vi "ConvertStringToArmSource.vi"(11 "Arm Source String":string) -> (3 "Arm Source":T1)   [LabVIEW 2012, in "Keithley-7001.lvlib"]
uses:
  Keithley-7001.lvlib
  Public/Controls/ArmSource.ctl
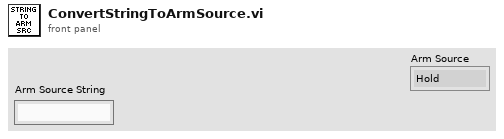
[diagram p1: front panel]
types:
  T1 = typedef "Keithley-7001.lvlib/ArmSource.ctl" = enum16{"Hold", "Immediate", "Manual", "Bus", "External"}
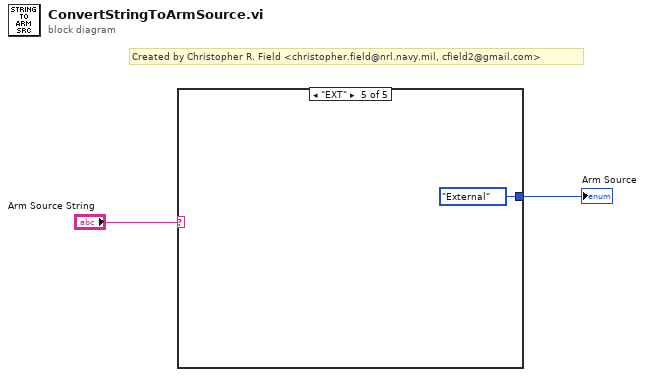
[diagram p0: block diagram]
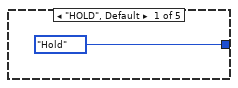
[diagram p2: hidden frame]
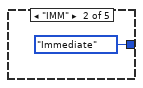
[diagram p3: hidden frame]
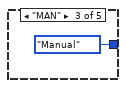
[diagram p4: hidden frame]
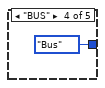
[diagram p5: hidden frame]
diagram:
  # "Created by Christopher R. Field <christopher.field@nrl.navy.mil, cfield2@gmail.com>"
  n1 = case shown="\"EXT\"" "Arm Source String" {
    tunnel: [ArmSource."Hold" ("Arm Source") ArmSource."Immediate" ("Arm Source") ArmSource."Manual" ("Arm Source") ArmSource."Bus" ("Arm Source") ArmSource."External" ("Arm Source")] -> w1
    frame "HOLD", Default {
    }
    frame "IMM" {
    }
    frame "MAN" {
    }
    frame "BUS" {
    }
    frame "EXT" {
    }
  }
  "Arm Source" <- w1
